vi "Load configuration.vi"(8 "error IO":errorcluster, 11 "Channel.lvclass":refnum<class "Channel.lvclass">) -> (0 "error IO 2":errorcluster, 2 "Initialization variables 2":T1={"Channel"=1, "ACS Simulated/Real"=FALSE, "Image path:"=path "E:/images/today", "Remote IP:"="200.131.64.49"}, 3 "Channel.lvclass 2":refnum<class "Channel.lvclass">)   [LabVIEW 2018, in "Channel.lvclass"]
uses:
  Channel.lvclass
  Channel.lvclass/Channel.ctl
  Configuration File/Configuration File.lvclass/Configuration File.ctl
  Configuration File/Configuration File.lvclass
  <vilib>/Utility/Data Type/NI_Data Type.lvlib
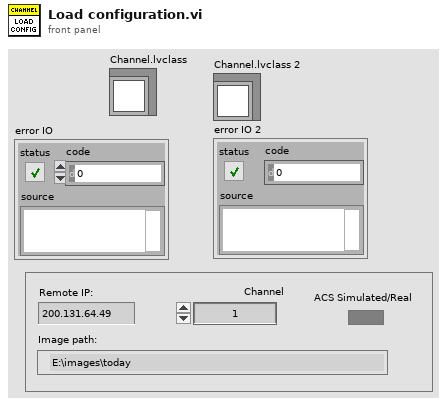
[diagram p1: front panel]
types:
  T1 = cluster{"Channel":u8, "ACS Simulated/Real":bool, "Image path:":path, "Remote IP:":string}
  T2 = typedef "NI_Data Type.lvlib/Data Type.ctl" = enum8{"Invalid Type", "Void", "I8", "I16", "I32", "I64", "U8", "U16", "U32", "U64", "Single Float", "Double Float", "Extended Float", "Single Complex", "Double Complex", "Extended Complex", "Enum U8", "Enum U16", "Enum U32", "Enum U64", "Single Float With Unit", "Double Float With Unit", "Extended Float With Unit", "Single Complex with Unit", "Double Complex with Unit", "Extended Complex with Unit", "Boolean", "String", "Path", "Picture", "Tag", "Array", "Cluster", "Variant", "LV Variant", "Waveform", "Timestamp", "Digital Waveform", "Digital Data", "ExpressData", "Refnum", "External Data", "VI", "Poly VI", "LabVIEW Class Instance", "Fixed Point"}
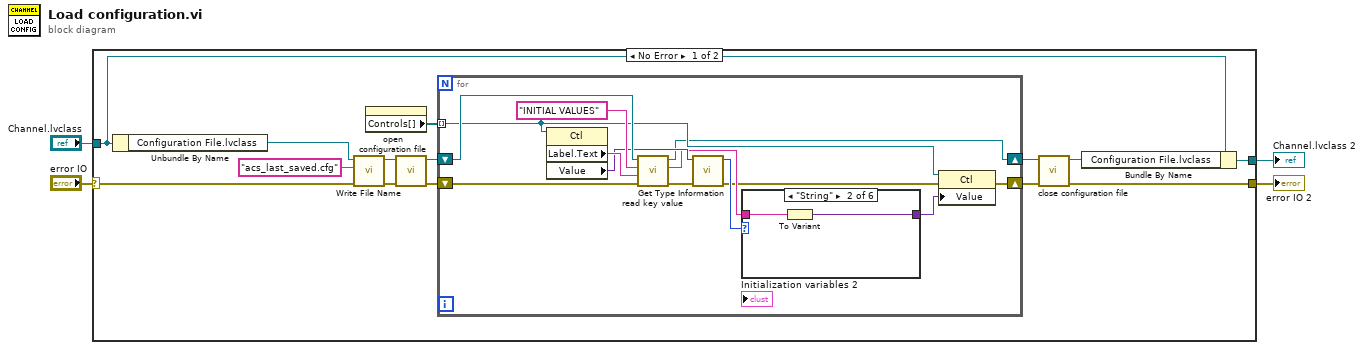
[diagram p0: block diagram]
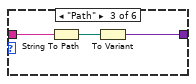
[diagram p3: hidden frame]
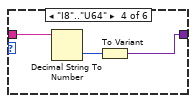
[diagram p4: hidden frame]
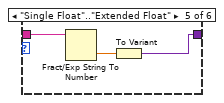
[diagram p5: hidden frame]
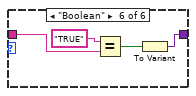
[diagram p6: hidden frame]
diagram:
  n1 = case shown="No Error" "error IO" {
    selector: "error IO" -> [w18 w48]
    tunnel: [w13 w48] -> w1
    tunnel: [w16 w47] -> w2
    tunnel: "Channel.lvclass" -> [w17 w47]
    frame No Error {
      n2 = Unbundle By Name(w17) -> ("Configuration File.lvclass"=w11:refnum<class "Configuration File.lvclass">)
      n3 = call "Write File Name.vi"("error in (no error)"=w18, "File Name"="acs_last_saved.cfg", "Configuration File in"=w11) -> ("error out"=w12:errorcluster, "Configuration File out"=w15:refnum<class "Configuration File.lvclass">)  [unwired: 7 in]
      n4 = property on="Initialization variables 2" class="Clust (strict)"() -> ("Controls[]"=w9:refnum<vi>[])  [unwired: 2 in, 2 out]
      n5 = call "open configuration file.vi"("error in (no error)"=w12, "Configuration File in"=w15) -> ("error out"=w7:errorcluster, "Configuration File out"=w8:refnum<class "Configuration File.lvclass">)  [unwired: 8 in]
      n6 = for {
        shift-right: [w21] -> w6
        shift-left: w8 -> [w29]
        shift-right: [w19] -> w5
        shift-left: w7 -> [w28]
        tunnel: w9 -> [w22] mode=indexing
        n7 = property class="Ctl"(reference=w22) -> ("Label.Text"=w31:string, "Value"=w27:variant)  [unwired: 1 in, 2 out]
        n8 = call "read key value.vi"("error in (no error)"=w28, "key"=w31, "section"="INITIAL VALUES", "Configuration File in"=w29) -> ("error out"=w26:errorcluster, "value"=w24:string, "Configuration File out"=w21:refnum<class "Configuration File.lvclass">)  [unwired: 5 in]
        n9 = call <vilib>:"Get Type Information.vi"("error in (no error)"=w26, "Variant"=w27) -> ("error out"=w20:errorcluster, "Type"=w25:T2)  [unwired: 5 in, 3 out]
        n10 = case shown="\"String\"" w25 {
          tunnel: w24 -> [_ w32 w35 w38 w41 w45]
          tunnel: [_ w33 w36 w39 w42 w46] -> w23
          frame "Invalid Type", Default {
          }
          frame "String" {
            n11 = To Variant(anything=w32) -> (Variant=w33:variant)
          }
          frame "Path" {
            n12 = String To Path(string=w35) -> (path=w34:path)
            n13 = To Variant(anything=w34) -> (Variant=w36:variant)
          }
          frame "I8".."U64" {
            n14 = Decimal String To Number(string=w38) -> (number=w37:i32)  [unwired: 2 in, 1 out]
            n15 = To Variant(anything=w37) -> (Variant=w39:variant)
          }
          frame "Single Float".."Extended Float" {
            n16 = Fract/Exp String To Number(string=w41) -> (number=w40:dbl)  [unwired: 3 in, 1 out]
            n17 = To Variant(anything=w40) -> (Variant=w42:variant)
          }
          frame "Boolean" {
            n18 = Equal?(x="TRUE", y=w45) -> (x = y?=w44:bool)
            n19 = To Variant(anything=w44) -> (Variant=w46:variant)
          }
        }
        n20 = property class="Ctl"(reference=w22, error in=w20, "Value"=w23) -> (error out=w19:errorcluster)  [unwired: 1 out]
      }
      n21 = call "close configuration file.vi"("error in (no error)"=w5, "Configuration File in"=w6) -> ("error out"=w13:errorcluster, "Configuration File out"=w14:refnum<class "Configuration File.lvclass">)  [unwired: 8 in]
      n22 = Bundle By Name(cluster=w17, "Configuration File.lvclass"=w14) -> (w16:refnum<class "Channel.lvclass">)
    }
    frame Error {
    }
  }
  "Channel.lvclass 2" <- w2
  "error IO 2" <- w1
